vi "Get Heartbeats.vi"(11 "CANopen in":refnum<class "CANopen.lvclass">) -> (2 "Heartbeats":T1(c390), 3 "CANopen out":refnum<class "CANopen.lvclass">)   [LabVIEW 2024, in "canopen.lvlib" / "CANopen.lvclass"]
uses:
  CANopen.lvclass
  CANopen.lvclass/CANopen.ctl
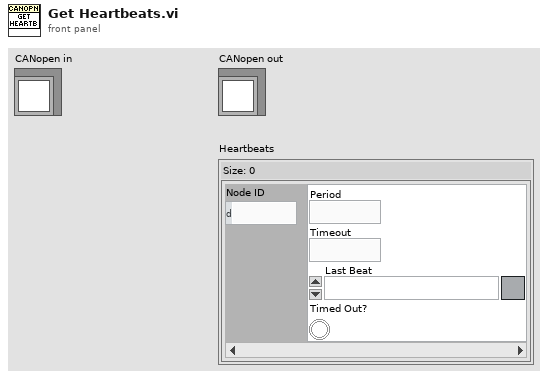
[diagram p1: front panel]
types:
  T1 = map{u8, cluster{"Period":u16, "Timeout":u16, "Last Beat":timestamp, "Timed Out?":bool}}
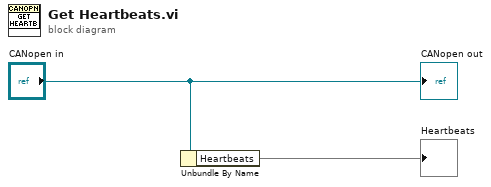
[diagram p0: block diagram]
diagram:
  n1 = Unbundle By Name("CANopen in") -> ("Heartbeats"=→"Heartbeats":T1)
  "CANopen out" <- "CANopen in"
